vi "Initialize Expansion Board UART connection.vi"(8 "error in (no error)":errorcluster) -> (0 "error out":errorcluster, 3 "SerialPortRef":T1)   [LabVIEW 2015]
uses:
  <vilib>/Rock Robotics/WPI/SerialPort/WPI_SerialPortRef.ctl
  <vilib>/Rock Robotics/WPI/SerialPort/WPI_SerialPort.ctl
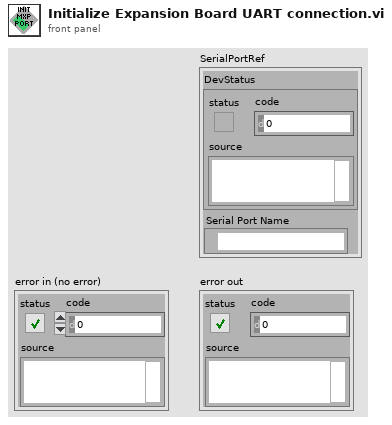
[diagram p1: front panel]
types:
  T1 = typedef "WPI_SerialPortRef.ctl" = cluster{"DevStatus":errorcluster, "Serial Port Name":refnum<visa-resource-name>}
  T2 = typedef "WPI_SerialPort.ctl" = enum16{"Onboard RS-232", "MXP TTL"}
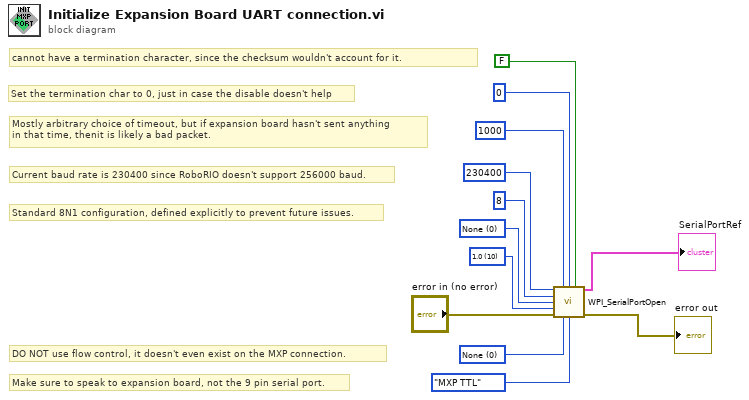
[diagram p0: block diagram]
diagram:
  w9 = u16 10 items=["1.0"=10, "1.5"=15, "2.0"=20] ("Stop Bits")
  w4 = u16 0 items=["None", "XON/XOFF", "RTS/CTS", "XON/XOFF & RTS/CTS", "DTR/DSR", "XON/XOFF & DTR/DSR"] ("Flow Control")
  w3 = u16 0 items=["None", "Odd", "Even", "Mark", "Space"] ("Parity")
  # "Make sure to speak to expansion board, not the 9 pin serial port."
  # "DO NOT use flow control, it doesn't even exist on the MXP connection."
  # "Standard 8N1 configuration, defined explicitly to prevent future issues."
  # "Current baud rate is 230400 since RoboRIO doesn't support 256000 baud."
  # "Mostly arbitrary choice of timeout, but if expansion board hasn't sent anything\nin that time, thenit is likely a bad packet."
  # "Set the termination char to 0, just in case the disable doesn't help"
  # "cannot have a termination character, since the checksum wouldn't account for it."
  n1 = call <vilib>:"WPI_SerialPortOpen.vi"("Baud Rate"=u32 230400, "Timeout Value (ms)"=u32 1000, "Termination Char (0xA = '\\n' = LF)"=u8 0 ("Termination Char (0xA = '\\n' = LF)"), "Enable Termination Char? (T)"=FALSE, "Data Bits"=u16 8, "Parity"=w3, "Stop Bits"=w9, "error in (no error)"="error in (no error)", "Flow Control"=w4, "Serial Port"=WPI_SerialPort."MXP TTL") -> ("SerialPortRef"=→"SerialPortRef":T1, "error out"=→"error out":errorcluster)  [unwired: 4 in]
